vi "Configure Glue Resirvoir.vi"(7 "Config Folder":path, 8 "error in (no error)":errorcluster, 11 "WorkTable Class in":refnum<class "WorkTable Class.lvclass">) -> (0 "error out":errorcluster, 3 "WorkTable Class out":refnum<class "WorkTable Class.lvclass">)   [LabVIEW 2011, in "WorkTable Class.lvclass"]
uses:
  WorkTable Class.lvclass
  Vec3d Class/Vec3d Class.lvclass
  <vilib>/Utility/config.llb/Read Key (U32).vi
  <vilib>/Utility/config.llb/Read Key (String).vi
  <vilib>/Utility/config.llb/NI_LVConfig.lvlib
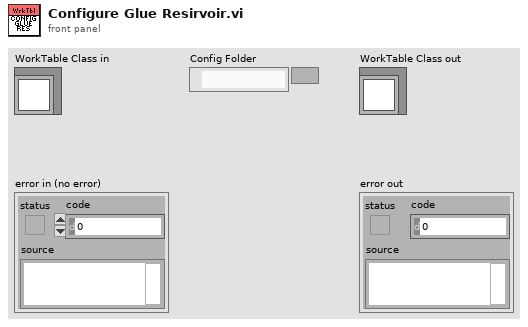
[diagram p1: front panel]
types:
  T1 = cluster{"Glue Reservoir Slots":cluster{"Reservoir State":enum16{"Empty", "Full", "Used"}, "Center":refnum<class "Vec3d Class.lvclass">}[], "Vacuum Channel":u8}
  T2 = cluster{"Reservoir State":enum16{"Empty", "Full", "Used"}, "Center":refnum<class "Vec3d Class.lvclass">}
  T3 = typedef "NI_LVConfig.lvlib/Config Data RefNum.ctl" = refnum<k1>
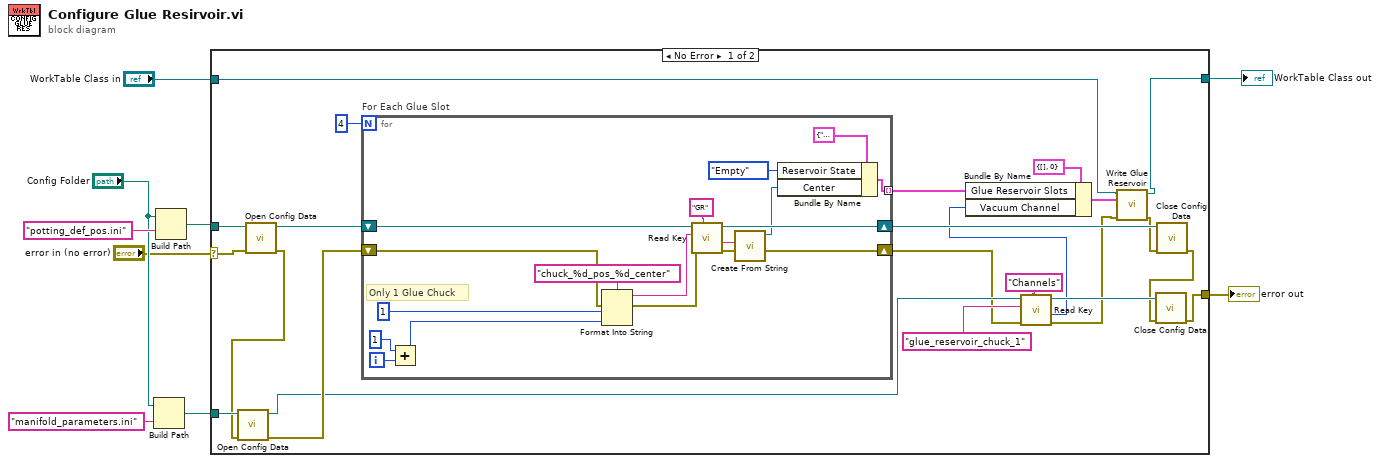
[diagram p0: block diagram]
diagram:
  n1 = Build Path(base path="Config Folder", name or relative path="manifold_parameters.ini") -> (appended path=w4:path)
  n2 = Build Path(base path="Config Folder", name or relative path="potting_def_pos.ini") -> (appended path=w5:path)
  n3 = case shown="No Error" "error in (no error)" {
    selector: "error in (no error)" -> [w32 w52]
    tunnel: [w18 w52] -> w2
    tunnel: [w16 w51] -> w1
    tunnel: "WorkTable Class in" -> [w17 w51]
    tunnel: w5 -> [w30 _]
    tunnel: w4 -> [w27 _]
    frame No Error {
      n4 = call <vilib>:"Open Config Data.vi"("error in (no error)"=w32, "configuration file path"=w30) -> ("error out"=w26:errorcluster, "refnum"=w29:T3)  [unwired: 7 in, 1 out]
      n5 = call <vilib>:"Open Config Data.vi"("error in (no error)"=w26, "configuration file path"=w27) -> ("error out"=w25:errorcluster, "refnum"=w23:T3)  [unwired: 7 in, 1 out]
      n6 = for "For Each Glue Slot" {
        N: 4 ("dimension size") -> [_]
        shift-right: [w47] -> w31
        shift-left: w29 -> [w48]
        shift-right: [w42] -> w21
        shift-left: w25 -> [w49]
        tunnel: [w45] -> w10 mode=indexing
        i -> [w46]
        # "Only 1 Glue Chuck"
        n7 = Add(x=1, y=w46) -> (x+y=w44:i32)
        n8 = Format Into String(format string="chuck_%d_pos_%d_center", error in=w49, 1, w44) -> (resulting string=w39:string, error out=w38:errorcluster)  [unwired: 1 in]
        n9 = call-poly <vilib>:"Read Key.vi"("section"="GR", "error in (no error)"=w38, "key"=w39, "refnum"=w48) -> ("error out"=w37:errorcluster, "value"=w36:string, "refnum out"=w47:T3)  [unwired: 4 in, 1 out]
        n10 = call "Create From String.vi"("error in (no error)"=w37, "Input String"=w36) -> ("error out"=w42:errorcluster, "Vec3d Class out"=w33:refnum<class "Vec3d Class.lvclass">)  [unwired: 8 in]
        n11 = Bundle By Name(cluster=T2 {"Reservoir State"=enum."Empty", "Center"=refnum} ("element"), "Reservoir State"=enum16{"Empty", "Full", "Used"}."Empty", "Center"=w33) -> (w45:T2)
      }
      n12 = call-poly <vilib>:"Read Key.vi"("section"="Channels", "error in (no error)"=w21, "key"="glue_reservoir_chuck_1" ("format string"), "refnum"=w23) -> ("error out"=w14:errorcluster, "value"=w12:u32, "refnum out"=w20:T3)  [unwired: 4 in, 1 out]
      n13 = Bundle By Name(cluster=T1 {"Glue Reservoir Slots"=[], "Vacuum Channel"=0} ("Glue Reservoir"), "Glue Reservoir Slots"=w10, "Vacuum Channel"=w12) -> (w11:T1)
      n14 = call-dynamic "Write Glue Reservoir.vi"("error in (no error)"=w14, "Glue Reservoir"=w11, "WorkTable Class in"=w17) -> ("error out"=w15:errorcluster, "WorkTable Class out"=w16:refnum<class "WorkTable Class.lvclass">)  [unwired: 7 in]
      n15 = call <vilib>:"Close Config Data.vi"("error in (no error)"=w15, "refnum"=w31) -> ("error out"=w19:errorcluster)  [unwired: 8 in, 1 out]
      n16 = call <vilib>:"Close Config Data.vi"("error in (no error)"=w19, "refnum"=w20) -> ("error out"=w18:errorcluster)  [unwired: 8 in, 1 out]
    }
    frame Error {
    }
  }
  "WorkTable Class out" <- w1
  "error out" <- w2
